vi "Initialize.vi"(8 "error in":errorcluster, 10 "shared resources":refnum<class "Shared Resources.lvclass">, 11 "Monitor Execution Unit Implementation in":refnum<class "Monitor Execution Unit.lvclass">) -> (0 "error out":errorcluster, 3 "Monitor Execution Unit Implementation out":refnum<class "Monitor Execution Unit.lvclass">)   [LabVIEW 2020, in "AIM ARINC 664 Engine.lvlib" / "Implementation.lvlib" / "Monitor Execution Unit.lvclass"]
uses:
  Monitor Execution Unit.lvclass
  Interfaces/Shared Resources/Shared Resources.lvclass
  Monitor Execution Unit.lvclass/Monitor Execution Unit.ctl
  <instrlib>/AIM GmbH/_AIM 664/bsp/Fdx Create Session (RX-Monitor).vi
  <instrlib>/AIM GmbH/_AIM 664/AIM664LV.lvlib
  <vilib>/Utility/SystemLogging/NI_SystemLogging.lvlib
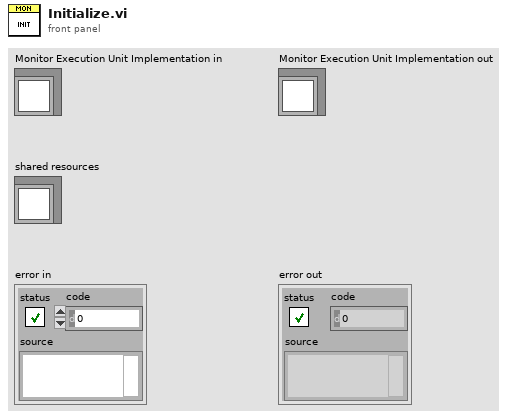
[diagram p1: front panel]
types:
  T1 = typedef "channel_settings_rx.ctl" = cluster{"Monitor Settings":T2, "Rx Board":u32, "Rx Port":u32}
  T2 = typedef "AIM664LV.lvlib/session_monitor_config.ctl" = cluster{"DefaultCronoMode":u32, "GlbMonBufferSizeIn":u32}
  T3 = typedef "monitor_queue_settings.ctl" = cluster{"TriggerPosition":u32, "CaptureMode":u32, "Strobe":u32, "MaxFileSize MB (1)":u32}
  T4 = typedef "loggingThreshold_types.ctl" = cluster{"Segmentation Threshold":dbl, "Disk Space Percentage":dbl, "Check Disk Space":bool, "Segment File":bool, "Segment Files By":u16}
  T5 = typedef "Frame Logging.lvlib/Log_Producer.ctl" = cluster{"Configured":bool, "message queue in":refnum<queue>, "StopNotification":refnum<notifier>}
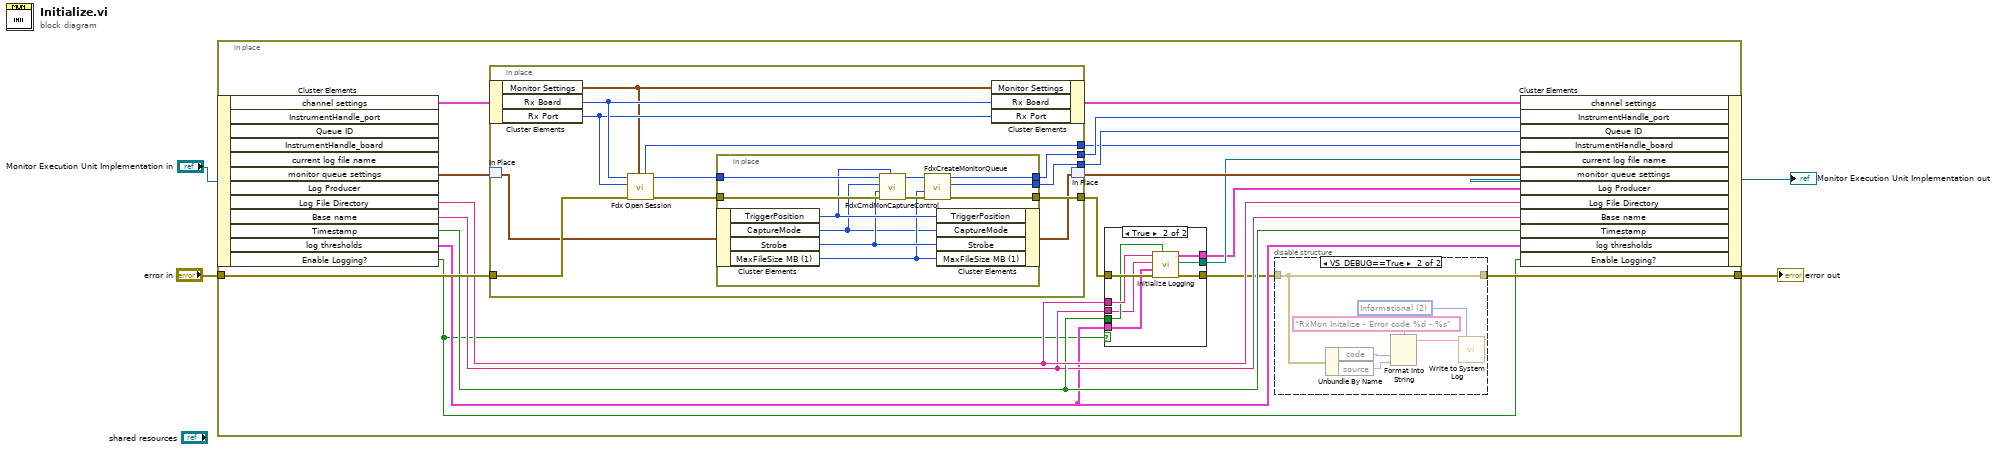
[diagram p0: block diagram]
diagram:
  n1 = in-place {
    in-place-border: "error in" -> [w20]
    in-place-border: [w6] -> w1
    n2 = in-place-cluster #1("Monitor Execution Unit Implementation in") -> ("channel settings"=w21:T1, "monitor queue settings"=w15:T3, "Log File Directory"=w11:string, "Base name"=w9:string, "Timestamp"=w10:bool, "log thresholds"=w8:T4, "Enable Logging?"=w5:bool)  [unwired: 5 out]
    n3 = in-place {
      in-place-border: w20 -> [w38]
      in-place-border: [w36] -> w18
      in-place-border: [w41] -> w17
      in-place-border: [w40] -> w22
      in-place-border: [w32] -> w16
      n4 = in-place-cluster #2(w21) -> ("Monitor Settings"=w35:T2, "Rx Board"=w39:u32, "Rx Port"=w37:u32)
      n5 = in-place-match #3(w15) -> (w33:T3)
      n6 = call-poly <instrlib>:"Fdx Open Session.vi"("MonitorConfig"=w35, "error in (no error)"=w38, "port"=w37, "board"=w39) -> ("error out"=w43:errorcluster, "InstrumentHandle_port out"=w42:u32, "InstrumentHandle_board out"=w32:u32)  [unwired: 2 in, 3 out]
      n7 = in-place {
        in-place-border: w42 -> [w54]
        in-place-border: [w50] -> w41
        in-place-border: [w49] -> w40
        in-place-border: w43 -> [w53]
        in-place-border: [w48] -> w36
        n8 = in-place-cluster #4(w33) -> ("TriggerPosition"=w47:u32, "CaptureMode"=w44:u32, "Strobe"=w46:u32, "MaxFileSize MB (1)"=w45:u32)
        n9 = call <instrlib>:"FdxCmdMonCaptureControl.vi"("TriggerPosition"=w47, "error in"=w53, "Strobe"=w46, "CaptureMode"=w44, "InstrumentHandle_port in"=w54) -> ("error out"=w52:errorcluster, "InstrumentHandle_port out"=w51:u32)  [unwired: 5 in]
        n10 = call <instrlib>:"FdxCreateMonitorQueue.vi"("error in (no error)"=w52, "MaxFileSize MB (1)"=w45, "InstrumentHandle_port in"=w51) -> ("error out"=w49:errorcluster, "QueueIdOut"=w48:u32, "InstrumentHandle_port out"=w50:u32)  [unwired: 5 in, 1 out]
        n11 = in-place-cluster #4("TriggerPosition"=w47, "CaptureMode"=w44, "Strobe"=w46, "MaxFileSize MB (1)"=w45) -> (w34:T3)
      }
      n12 = in-place-cluster #2("Monitor Settings"=w35, "Rx Board"=w39, "Rx Port"=w37) -> (w19:T1)
      n13 = in-place-match #3(w34) -> (w14:T3)
    }
    n14 = case shown="True" w5 {
      tunnel: w22 -> [w23 w31]
      tunnel: [_ w30] -> w13
      tunnel: [_ w29] -> w12
      tunnel: w11 -> [_ w28]
      tunnel: w10 -> [_ w27]
      tunnel: w9 -> [_ w26]
      tunnel: w8 -> [_ w25]
      tunnel: [w23 w24] -> w7
      frame False {
      }
      frame True {
        n15 = call "Initialize Logging.vi"("Timestamp"=w27, "error in"=w31, "log thresholds"=w25, "Base name"=w26, "Log File Directory"=w28) -> ("error out"=w24:errorcluster, "File path out"=w30:path, "Log Producer out"=w29:T5)  [unwired: 4 in]
      }
    }
    n16 = disable-structure shown="VS_DEBUG==True" {
      disable-tunnel: w7 -> [w55 w56]
      disable-tunnel: [w55 w56] -> w6
      frame condition #0 (active) {
      }
      frame condition #1 {
        w59 = 2 items=["Error", "Warning", "Informational"] ("severity")
        n17 = Unbundle By Name(w56) -> ("code"=w58:i32, "source"=w57:string)
        n18 = Format Into String(format string="RxMon Initalize - Error code %d - %s", w58, w57) -> (resulting string=w60:string)  [unwired: 2 in, 1 out]
        n19 = call <vilib>:"Write to System Log.vi"("severity"=w59, "message"=w60) -> ()  [unwired: 9 in, 1 out]
      }
    }
    n20 = in-place-cluster #1("channel settings"=w19, "InstrumentHandle_port"=w17, "Queue ID"=w18, "InstrumentHandle_board"=w16, "current log file name"=w13, "monitor queue settings"=w14, "Log Producer"=w12, "Log File Directory"=w11, "Base name"=w9, "Timestamp"=w10, "log thresholds"=w8, "Enable Logging?"=w5) -> (→"Monitor Execution Unit Implementation out":refnum<class "Monitor Execution Unit.lvclass">)
  }
  "error out" <- w1
